vi "UpdateFPReply.vi"(1 "error in (no error)":errorcluster, 2 "Reply":string, 3 "Sent":string, 4 "method":string) -> (0 "Log":T1)   [LabVIEW 2012]
uses:
  <userlib>/ROSforLV/ROS/Code/Console/Servers/ServerSubs/ROSLog.ctl
  <userlib>/ROSforLV/ROS/Code/_ROSDefinition.vi
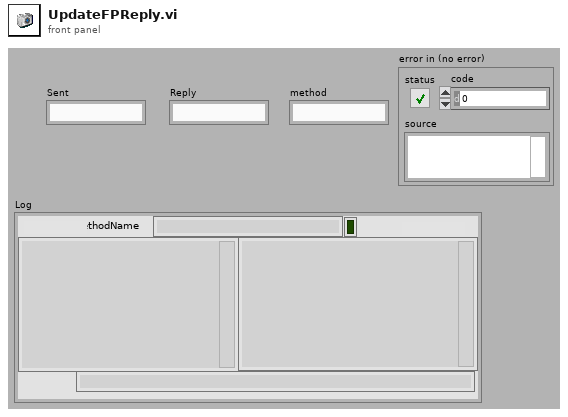
[diagram p1: front panel]
types:
  T1 = typedef "ROSLog.ctl" = cluster{"Sent":string, "Reply":string, "MethodName":string, "success":bool, "Dir1":string, "Dir2":string, "Time Stamp":string, "error":errorcluster, "Preamble":string, "Midamble":string, "Postamble":string}
  T2 = cluster{"Sent":string, "Reply":string, "method":string, bool, "element":string, "element":string, "Current Time":string, "error in (no error)":errorcluster, string, string, string}
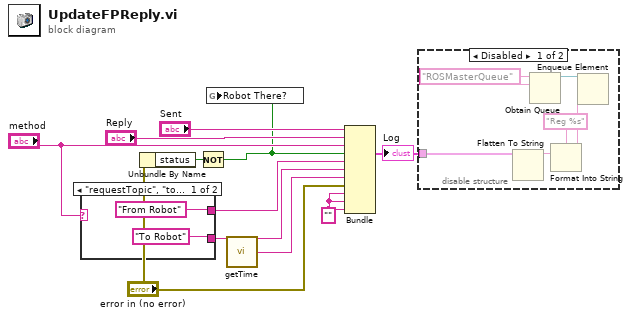
[diagram p0: block diagram]
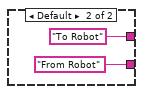
[diagram p2: hidden frame]
diagram:
  w1 = ""
  n1 = case shown="\"requestTopic\", \"topicReply\"" "method" {
    tunnel: ["From Robot" ("element") "To Robot" ("element")] -> w8
    tunnel: ["To Robot" ("element") "From Robot" ("element")] -> w7
    frame "requestTopic", "topicReply" {
    }
    frame Default {
    }
  }
  n2 = Unbundle By Name("error in (no error)") -> ("status"=w3:bool)
  n3 = Not(x=w3) -> (.not. x?=w2:bool)
  n4 = global write "_ROSDefinition.vi" "Robot There?"(w2) -> ()
  n5 = call <userlib>:"getTime.vi"() -> ("Current Time"=w6:string)  [unwired: 1 in]
  n6 = Bundle("Sent"="Sent", "Reply"="Reply", "method"="method", w2, "element"=w8, "element"=w7, "Current Time"=w6, "error in (no error)"="error in (no error)", w1, w1, w1) -> (w11:T2)  [unwired: 1 in]
  "Log" <- w11
  n7 = disable-structure shown="Disabled" {
    disable-tunnel: w11 -> [w19 _]
    frame Disabled {
      w16 = "ROSMasterQueue" ("name (unnamed)")
      n8 = Flatten To String(anything=w19) -> (data string=w20:string)  [unwired: 3 in, 2 out]
      n9 = Obtain Queue(name (unnamed)=w16, element data type=w16) -> (queue out=w17:refnum<queue>)  [unwired: 3 in, 2 out]
      n10 = Format Into String(format string="Reg %s" ("element"), w20) -> (resulting string=w21:string)  [unwired: 2 in, 1 out]
      n11 = Enqueue Element(queue=w17, element=w21) -> ()  [unwired: 2 in, 3 out]
    }
    frame Enabled {
    }
  }
